vi "Configure Data Replay Loops.vi"(6 "DataReplayLoops":T1[](array[typedef]), 8 "error in (no error)":errorcluster, 10 "FPGA Session":u32, 11 "FPGA Interface Base in":refnum<class "FPGA Interface Base.lvclass">) -> (0 "error out":errorcluster, 2 "FPGA Session dup":u32, 3 "FPGA Interface Base out":refnum<class "FPGA Interface Base.lvclass">)   [LabVIEW 2011, in "Engine Sim RT.lvlib"]
uses:
  Engine Sim RT.lvlib
  <userlib>/_FPGA Interface Advanced Tools/FPGA Interface Base/FPGA Interface Base.lvclass
  Shared/DataReplayLoopConfig.ctl
  Shared/DataReplayConfig.ctl
  <vilib>/rvi/DataTransferAndStorage/Container/Common/niFpgaDataTypeControl.ctl
  <userlib>/_FPGA Interface Advanced Tools/FPGA Interface Base/FPGA Interface Base.lvclass/FPGA Interface Base.ctl
  <userlib>/_FPGA Interface Advanced Tools/FPGA Interface Wrapper/NiFPGA Write Array - I16.vi
  <userlib>/_FPGA Interface Advanced Tools/FPGA Interface Wrapper/NiFPGA Write - Boolean.vi
  <userlib>/_FPGA Interface Advanced Tools/FPGA Interface Wrapper/NiFPGA Read - Boolean.vi
  <userlib>/_FPGA Interface Advanced Tools/FPGA Interface Wrapper/NiFPGA Write - U16.vi
  <vilib>/Utility/error.llb/Error Cluster From Error Code.vi
  <userlib>/_FPGA Interface Advanced Tools/FPGA Interface Base/FPGA Write By Name - U32.vi
  <userlib>/_FPGA Interface Advanced Tools/FPGA Interface Base/FPGA Write By Name - I8.vi
  <userlib>/_FPGA Interface Advanced Tools/FPGA Interface Base/FPGA Write By Name - I32.vi
  <userlib>/_FPGA Interface Advanced Tools/FPGA Interface Base/FPGA Write By Name - U64.vi
  <userlib>/_FPGA Interface Advanced Tools/FPGA Interface Base/FPGA Write By Name - Boolean.vi
  <userlib>/_FPGA Interface Advanced Tools/FPGA Interface Wrapper/FPGA Interface Wrapper.lvlib
  Engine Simulation Shared.lvlib
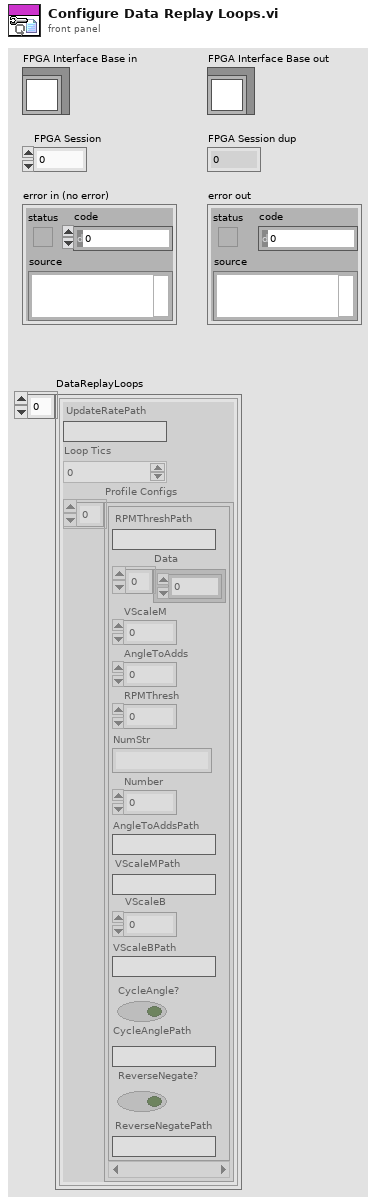
[diagram p1: front panel]
types:
  T1 = typedef "Engine Simulation Shared.lvlib/DataReplayLoopConfig.ctl" = cluster{"UpdateRatePath":string, "Loop Tics":u32, "Profile Configs":T2[]}
  T2 = typedef "Engine Simulation Shared.lvlib/DataReplayConfig.ctl" = cluster{"RPMThreshPath":string, "Data":i16[], "VScaleM":u32, "AngleToAdds":u32, "RPMThresh":u64, "NumStr":string, "Number":i8, "AngleToAddsPath":string, "VScaleMPath":string, "VScaleB":i32, "VScaleBPath":string, "CycleAngle?":bool, "CycleAnglePath":string, "ReverseNegate?":bool, "ReverseNegatePath":string}
  T3 = typedef "niFpgaDataTypeControl.ctl" = enum32{"Boolean", "I8", "I16", "I32", "I64", "U8", "U16", "U32", "U64", "FXP", "CustomControl"}
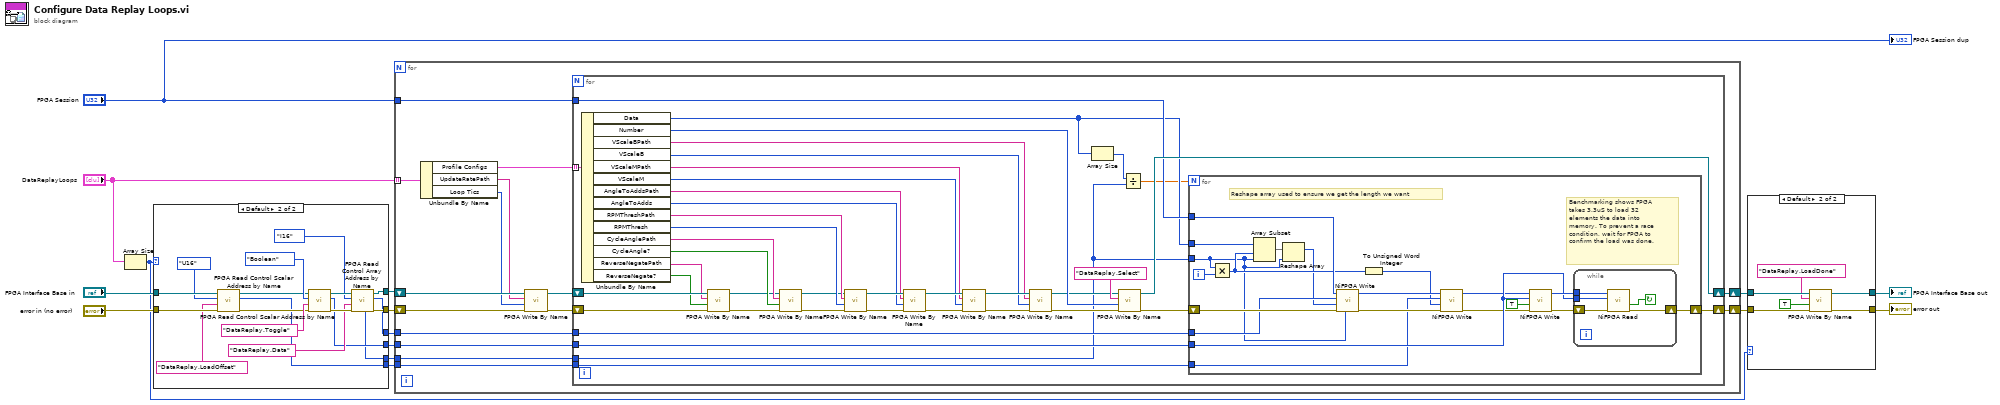
[diagram p0: block diagram]
diagram:
  n1 = Array Size(array="DataReplayLoops") -> (size(s)=w3:i32)
  n2 = case shown="Default" w3 {
    tunnel: "error in (no error)" -> [w16 w24]
    tunnel: "FPGA Interface Base in" -> [w17 w23]
    tunnel: [w17 w33] -> w11
    tunnel: [w16 w32] -> w10
    tunnel: [_ w27] -> w9
    tunnel: [_ w26] -> w8
    tunnel: [_ w25] -> w2
    tunnel: [_ w18] -> w1
    frame 0 {
    }
    frame Default {
      n3 = call <userlib>:"FPGA Read Control Scalar Address by Name.vi"("error in (no error)"=w24, "Name"="DataReplay.LoadOffset" ("string"), "Data Type"=niFpgaDataTypeControl."U16", "FPGA Interface Base in"=w23) -> ("error out"=w20:errorcluster, "Address"=w18:u32, "FPGA Interface Base out"=w19:refnum<class "FPGA Interface Base.lvclass">)  [unwired: 4 in, 1 out]
      n4 = call <userlib>:"FPGA Read Control Scalar Address by Name.vi"("error in (no error)"=w20, "Name"="DataReplay.Toggle" ("string"), "Data Type"=niFpgaDataTypeControl."Boolean", "FPGA Interface Base in"=w19) -> ("error out"=w34:errorcluster, "Address"=w27:u32, "FPGA Interface Base out"=w35:refnum<class "FPGA Interface Base.lvclass">)  [unwired: 4 in, 1 out]
      n5 = call <userlib>:"FPGA Read Control Array Address by Name.vi"("error in (no error)"=w34, "Name"="DataReplay.Data" ("string"), "Data Type"=niFpgaDataTypeControl."I16", "FPGA Interface Base in"=w35) -> ("error out"=w32:errorcluster, "Address"=w26:u32, "FPGA Interface Base out"=w33:refnum<class "FPGA Interface Base.lvclass">, "Num Elements"=w25:u32)  [unwired: 3 in, 1 out]
    }
  }
  n6 = for {
    tunnel: "DataReplayLoops" -> [w50] mode=indexing
    shift-right: [w39] -> w15
    shift-left: w10 -> [w48]
    shift-right: [w40] -> w6
    shift-left: w11 -> [w47]
    tunnel: "FPGA Session" -> [w43]
    tunnel: w9 -> [w42]
    tunnel: w8 -> [w41]
    tunnel: w2 -> [w37]
    tunnel: w1 -> [w36]
    n7 = Unbundle By Name(w50) -> ("Profile Configs"=w49:T2[], "UpdateRatePath"=w38:string, "Loop Tics"=w46:u32)
    n8 = call-poly <userlib>:"FPGA Write By Name.vi"("error in (no error)"=w48, "Value"=w46, "Control"=w38, "FPGA Session In"=w47) -> ("error out"=w45:errorcluster, "FPGA Session Out"=w44:refnum<class "FPGA Interface Base.lvclass">)  [unwired: 6 in]
    n9 = for {
      tunnel: w49 -> [w90] mode=indexing
      shift-right: [w73] -> w39
      shift-left: w45 -> [w89]
      shift-right: [w77] -> w40
      shift-left: w44 -> [w54]
      tunnel: w43 -> [w76]
      tunnel: w42 -> [w74]
      tunnel: w41 -> [w75]
      tunnel: w37 -> [w57]
      tunnel: w36 -> [w56]
      n10 = Unbundle By Name(w90) -> ("Data"=w60:i16[], "Number"=w79:i8, "VScaleBPath"=w66:string, "VScaleB"=w65:i32, "VScaleMPath"=w70:string, "VScaleM"=w82:u32, "AngleToAddsPath"=w71:string, "AngleToAdds"=w85:u32, "RPMThreshPath"=w72:string, "RPMThresh"=w88:u64, "CycleAnglePath"=w61:string, "CycleAngle?"=w62:bool, "ReverseNegatePath"=w52:string, "ReverseNegate?"=w51:bool)
      n11 = call-poly <userlib>:"FPGA Write By Name.vi"("error in (no error)"=w89, "Value"=w51, "Control"=w52, "FPGA Session In"=w54) -> ("error out"=w55:errorcluster, "FPGA Session Out"=w53:refnum<class "FPGA Interface Base.lvclass">)  [unwired: 6 in]
      n12 = call-poly <userlib>:"FPGA Write By Name.vi"("error in (no error)"=w55, "Value"=w62, "Control"=w61, "FPGA Session In"=w53) -> ("error out"=w64:errorcluster, "FPGA Session Out"=w63:refnum<class "FPGA Interface Base.lvclass">)  [unwired: 6 in]
      n13 = call-poly <userlib>:"FPGA Write By Name.vi"("error in (no error)"=w64, "Value"=w88, "Control"=w72, "FPGA Session In"=w63) -> ("error out"=w86:errorcluster, "FPGA Session Out"=w87:refnum<class "FPGA Interface Base.lvclass">)  [unwired: 6 in]
      n14 = call-poly <userlib>:"FPGA Write By Name.vi"("error in (no error)"=w86, "Value"=w85, "Control"=w71, "FPGA Session In"=w87) -> ("error out"=w83:errorcluster, "FPGA Session Out"=w84:refnum<class "FPGA Interface Base.lvclass">)  [unwired: 6 in]
      n15 = call-poly <userlib>:"FPGA Write By Name.vi"("error in (no error)"=w83, "Value"=w82, "Control"=w70, "FPGA Session In"=w84) -> ("error out"=w81:errorcluster, "FPGA Session Out"=w68:refnum<class "FPGA Interface Base.lvclass">)  [unwired: 6 in]
      n16 = call-poly <userlib>:"FPGA Write By Name.vi"("error in (no error)"=w81, "Value"=w65, "Control"=w66, "FPGA Session In"=w68) -> ("error out"=w69:errorcluster, "FPGA Session Out"=w67:refnum<class "FPGA Interface Base.lvclass">)  [unwired: 6 in]
      n17 = Array Size(array=w60) -> (size(s)=w59:i32)
      n18 = call-poly <userlib>:"FPGA Write By Name.vi"("error in (no error)"=w69, "Value"=w79, "Control"="DataReplay.Select" ("string"), "FPGA Session In"=w67) -> ("error out"=w78:errorcluster, "FPGA Session Out"=w77:refnum<class "FPGA Interface Base.lvclass">)  [unwired: 6 in]
      n19 = Divide(x=w59, y=w57) -> (x/y=w58:dbl)
      n20 = for {
        N: w58 -> [_]
        shift-right: [w100] -> w73
        shift-left: w78 -> [w110]
        tunnel: w76 -> [w109]
        tunnel: w75 -> [w108]
        tunnel: w74 -> [w102]
        tunnel: w60 -> [w106]
        tunnel: w57 -> [w91]
        tunnel: w56 -> [w94]
        i -> [w104]
        # "Reshape array used to ensure we get the length we want"
        # "Benchmarking shows FPGA takes 3.3uS to load 32 elements the data into memory. To prevent a race condition, wait for FPGA to confirm the load was done."
        n21 = Multiply(x=w91, y=w104) -> (x*y=w95:u32)
        n22 = Array Subset(array=w106, index=w95, length=w91) -> (w105:i16[])
        n23 = Reshape Array(w105, w91) -> (w92:i16[])
        n24 = call-poly <userlib>:"NiFPGA Write.vi"("Size"=w91, "error in (no error)"=w110, "Array"=w92, "Control"=w108, "Session"=w109) -> ("error out"=w96:errorcluster, "Session Out"=w99:u32)  [unwired: 5 in]
        n25 = To Unsigned Word Integer(number=w95) -> (unsigned 16bit integer=w93:u16)
        n26 = call-poly <userlib>:"NiFPGA Write.vi"("error in (no error)"=w96, "Value"=w93, "Control"=w94, "Session"=w99) -> ("error out"=w97:errorcluster, "Session Out"=w98:u32)  [unwired: 6 in]
        n27 = call-poly <userlib>:"NiFPGA Write.vi"("error in (no error)"=w97, "Boolean"=TRUE, "Control"=w102, "Session"=w98) -> ("error out"=w101:errorcluster, "Session Out"=w103:u32)  [unwired: 6 in]
        n28 = while {
          tunnel: w103 -> [w115]
          tunnel: w102 -> [w114]
          shift-right: [w111] -> w100
          shift-left: w101 -> [w113]
          stop <- w112 continue-if-true
          n29 = call-poly <userlib>:"NiFPGA Read.vi"("error in (no error)"=w113, "Indicator"=w114, "Session"=w115) -> ("error out"=w111:errorcluster, "Boolean"=w112:bool)  [unwired: 6 in, 1 out]
        }
      }
    }
  }
  n30 = case shown="Default" w3 {
    tunnel: w15 -> [w116 w123]
    tunnel: [w116 w122] -> w7
    tunnel: w6 -> [w117 w121]
    tunnel: [w117 w120] -> w5
    frame 0 {
    }
    frame Default {
      n31 = call-poly <userlib>:"FPGA Write By Name.vi"("error in (no error)"=w123, "Value"=TRUE ("Boolean"), "Control"="DataReplay.LoadDone" ("string"), "FPGA Session In"=w121) -> ("error out"=w122:errorcluster, "FPGA Session Out"=w120:refnum<class "FPGA Interface Base.lvclass">)  [unwired: 6 in]
    }
  }
  "FPGA Interface Base out" <- w5
  "error out" <- w7
  "FPGA Session dup" <- "FPGA Session"
